vi "右工位判定.vi"(7 "Result":refnum<vi>, 10 "右工位判定":T1, 11 "XY曲线":cluster{"X":dbl[], "Y":dbl[]}[](array[cluster])) -> (2 "大小":i32, 3 "OK？":bool)   [LabVIEW 2020]
uses:
  Global_Variable/Global.vi
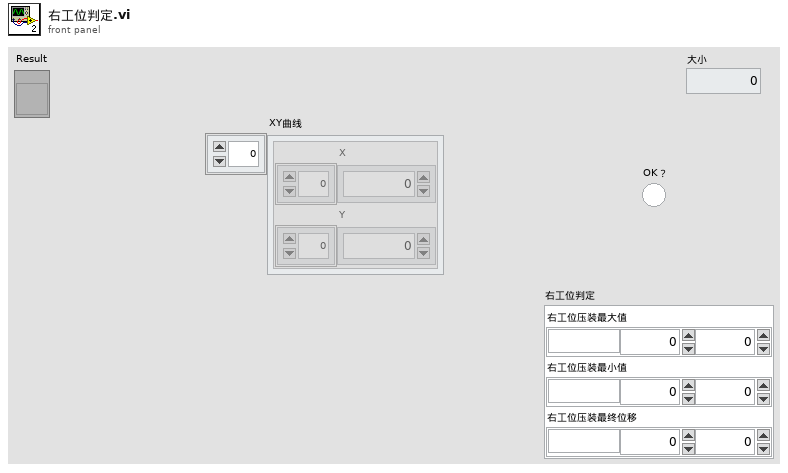
[diagram p1: front panel]
types:
  T1 = cluster{"右工位压装最大值":cluster{"单位":string, "下限":dbl, "上限":dbl}, "右工位压装最小值":cluster{"单位":string, "下限":dbl, "上限":dbl}, "右工位压装最终位移":cluster{"单位":string, "下限":dbl, "上限":dbl}}
  T2 = cluster{"X ":cluster{"单位":string, "下限":dbl, "上限":dbl}, "Y":cluster{"单位":string, "下限":dbl, "上限":dbl}}
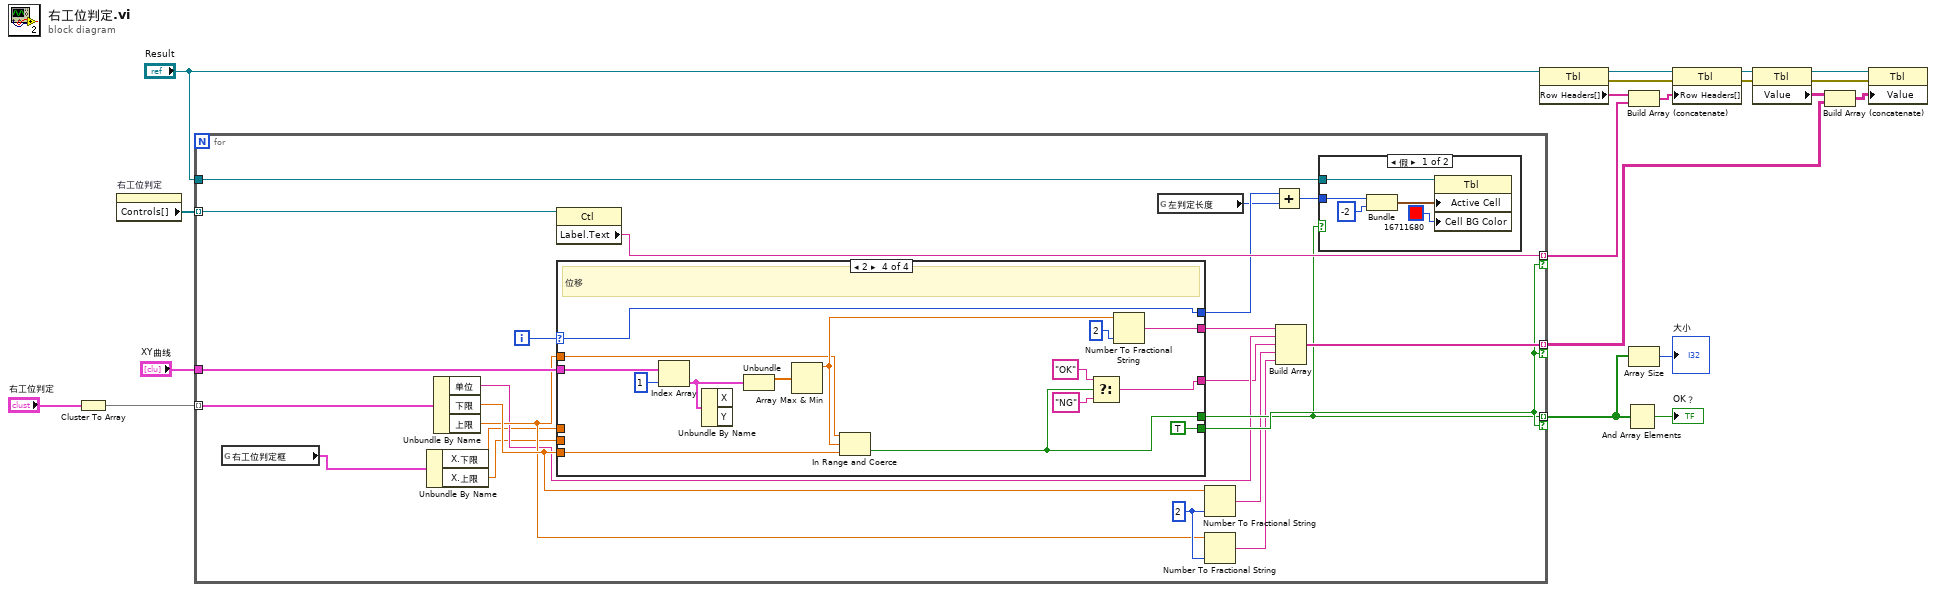
[diagram p0: block diagram]
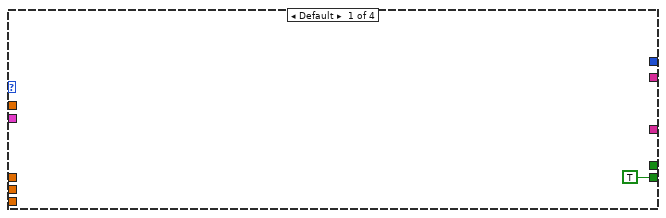
[diagram p3: hidden frame]
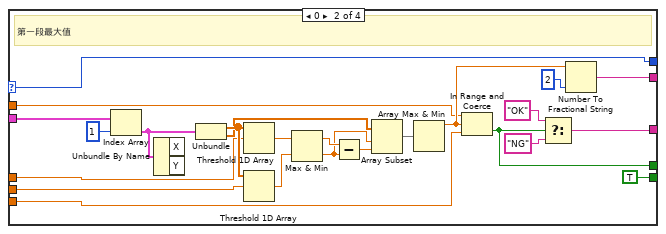
[diagram p4: hidden frame]
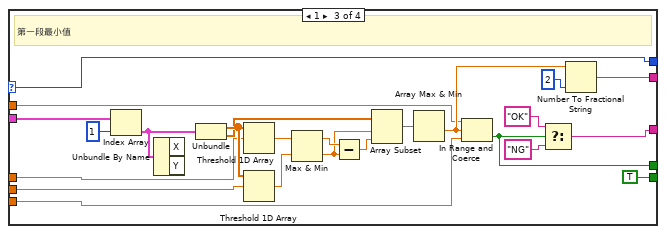
[diagram p5: hidden frame]
diagram:
  n1 = Cluster To Array(cluster="右工位判定") -> (array=w20:cluster{"单位":string, "下限":dbl, "上限":dbl}[])
  n2 = property on="右工位判定" class="Clust (严格)"() -> ("Controls[]"=w1:refnum<vi>[])  [unwired: 2 in, 2 out]
  n3 = for {
    tunnel: w20 -> [w43] mode=indexing
    tunnel: w1 -> [w41] mode=indexing
    tunnel: "XY曲线" -> [w40]
    tunnel: [w32] -> w4 mode=indexing if=w33
    tunnel: [w36] -> w6 mode=indexing if=w33
    tunnel: [w35] -> w8 mode=indexing if=w33
    tunnel: "Result" -> [w34]
    i -> [w42]
    w39 = i16 2 ("精度(6)")
    n4 = global read "Global.vi" "右工位判定框"() -> (w21:T2)
    n5 = Unbundle By Name(w21) -> ("X.下限"=w26:dbl, "X.上限"=w25:dbl)
    n6 = Unbundle By Name(w43) -> ("单位"=w30:string, "下限"=w38:dbl, "上限"=w37:dbl)
    n7 = property class="Ctl"(reference=w41) -> ("Label.Text"=w35:string)  [unwired: 1 in, 2 out]
    n8 = case shown="2" w42 {
      selector: w42 -> [_ w54 w78 w102]
      tunnel: w40 -> [_ w73 w97 w112]
      tunnel: [_ w70 w94 w109] -> w29
      tunnel: [_ w69 w93 w108] -> w32
      tunnel: w38 -> [_ w53 w77 w100]
      tunnel: w37 -> [_ w52 w76 w99]
      tunnel: [TRUE TRUE TRUE TRUE] -> w33
      tunnel: [_ w55 w79 w104] -> w31
      tunnel: [_ w54 w78 w102] -> w24
      tunnel: w26 -> [_ w51 w75 _]
      tunnel: w25 -> [_ w50 w74 _]
      frame Default {
      }
      frame 0 {
        # "第一段最大值"
        n9 = Index Array(array=w73, index=1 ("索引")) -> (element=w64:cluster{"X":dbl[], "Y":dbl[]})
        n10 = Unbundle By Name(w64) -> ()  [unwired: 2 out]
        n11 = Unbundle(w64) -> ("X"=w63:dbl[], "Y"=w60:dbl[])
        n12 = Threshold 1D Array(2:w51, 3:w63) -> (0:w67:dbl)  [unwired: 1 in]
        n13 = Threshold 1D Array(2:w50, 3:w63) -> (0:w66:dbl)  [unwired: 1 in]
        n14 = Max & Min(x=w67, y=w66) -> (max(x,y)=w65:dbl, min(x,y)=w61:dbl)
        n15 = Subtract(x=w65, y=w61) -> (x-y=w62:dbl)
        n16 = Array Subset(array=w60, index=w61, length=w62) -> (w59:dbl[])
        n17 = Array Max & Min(array=w59) -> (max value=w56:dbl)  [unwired: 3 out]
        n18 = In Range and Coerce(upper limit=w52, x=w56, lower limit=w53) -> (In Range?=w69:bool)  [unwired: 1 out]
        n19 = Select(t="OK", s=w69, f="NG") -> (s? t:f=w70:string)
        n20 = Number To Fractional String(number=w56, precision (6)=i16 2 ("精度(6)")) -> (F-format string=w55:string)  [unwired: 2 in]
      }
      frame 1 {
        # "第一段最小值"
        n21 = Index Array(array=w97, index=1 ("索引")) -> (element=w88:cluster{"X":dbl[], "Y":dbl[]})
        n22 = Unbundle By Name(w88) -> ()  [unwired: 2 out]
        n23 = Unbundle(w88) -> ("X"=w87:dbl[], "Y"=w84:dbl[])
        n24 = Threshold 1D Array(2:w75, 3:w87) -> (0:w91:dbl)  [unwired: 1 in]
        n25 = Threshold 1D Array(2:w74, 3:w87) -> (0:w90:dbl)  [unwired: 1 in]
        n26 = Max & Min(x=w91, y=w90) -> (max(x,y)=w89:dbl, min(x,y)=w85:dbl)
        n27 = Subtract(x=w89, y=w85) -> (x-y=w86:dbl)
        n28 = Array Subset(array=w84, index=w85, length=w86) -> (w83:dbl[])
        n29 = Array Max & Min(array=w83) -> (min value=w80:dbl)  [unwired: 3 out]
        n30 = In Range and Coerce(upper limit=w76, x=w80, lower limit=w77) -> (In Range?=w93:bool)  [unwired: 1 out]
        n31 = Select(t="OK", s=w93, f="NG") -> (s? t:f=w94:string)
        n32 = Number To Fractional String(number=w80, precision (6)=i16 2 ("精度(6)")) -> (F-format string=w79:string)  [unwired: 2 in]
      }
      frame 2 {
        # "位移"
        n33 = Index Array(array=w112, index=1 ("索引")) -> (element=w106:cluster{"X":dbl[], "Y":dbl[]})
        n34 = Unbundle By Name(w106) -> ()  [unwired: 2 out]
        n35 = Unbundle(w106) -> ("X"=w98:dbl[])  [unwired: 1 out]
        n36 = Array Max & Min(array=w98) -> (max value=w103:dbl)  [unwired: 3 out]
        n37 = In Range and Coerce(upper limit=w99, x=w103, lower limit=w100) -> (In Range?=w108:bool)  [unwired: 1 out]
        n38 = Select(t="OK", s=w108, f="NG") -> (s? t:f=w109:string)
        n39 = Number To Fractional String(number=w103, precision (6)=i16 2 ("精度(6)")) -> (F-format string=w104:string)  [unwired: 2 in]
      }
    }
    n40 = global read "Global.vi" "左判定长度"() -> (w22:i32)
    n41 = Number To Fractional String(number=w38, precision (6)=w39) -> (F-format string=w28:string)  [unwired: 2 in]
    n42 = Number To Fractional String(number=w37, precision (6)=w39) -> (F-format string=w27:string)  [unwired: 2 in]
    n43 = Add(x=w24, y=w22) -> (x+y=w23:i32)
    n44 = Build Array(w31, w30, w29, w28, w27) -> (w36:string[])
    n45 = case shown="假" w32 {
      tunnel: w34 -> [w48 _]
      tunnel: w23 -> [w44 _]
      frame False {
        n46 = Bundle(w44, -2) -> (w46:cluster{i32, i32})  [unwired: 1 in]
        n47 = property class="Tbl"(reference=w48, "Active Cell"=w46, "Cell BG Color"=u32 16711680 ("活动单元格:单元格背景色")) -> ()  [unwired: 1 in, 2 out]
      }
      frame True {
      }
    }
  }
  n48 = property class="Tbl"(reference="Result") -> (reference out=w10:refnum<vi>, error out=w15:errorcluster, "Row Headers[]"=w7:string[])  [unwired: 1 in]
  n49 = And Array Elements(Boolean array=w4) -> (logical AND=→"OK？":bool)
  n50 = Build Array (concatenate)(w7, w8) -> (w9:string[])
  n51 = Array Size(array=w4) -> (size(s)=→"大小":i32)
  n52 = property class="Tbl"(reference=w10, error in=w15, "Row Headers[]"=w9) -> (reference out=w11:refnum<vi>, error out=w14:errorcluster)
  n53 = property class="Tbl"(reference=w11, error in=w14) -> (reference out=w12:refnum<vi>, error out=w13:errorcluster, "Value"=w16:string[][])
  n54 = Build Array (concatenate)(w16, w6) -> (w17:string[][])
  n55 = property class="Tbl"(reference=w12, error in=w13, "Value"=w17) -> ()  [unwired: 2 out]
